vi "Set Password.vi"(8 "error in (no error)":errorcluster, 9 "New password":string, 10 "ProjectItem Refnum":refnum<vi>, 11 "Build in":refnum<class "NI_AB_API_Build.lvclass">) -> (0 "error out":errorcluster, 3 "Build out":refnum<class "NI_AB_API_Build.lvclass">)   [LabVIEW 2020, in "NI_AB_API_Build.lvclass"]
uses:
  <vilib>/AppBuilder/AB_API/Build/NI_AB_API_Build.lvclass
  <vilib>/AppBuilder/AB_API/Build/NI_AB_API_Build.lvclass/NI_AB_API_Build.ctl
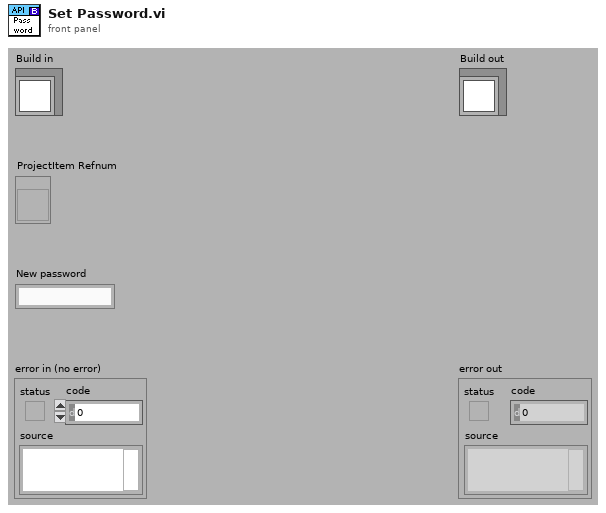
[diagram p1: front panel]
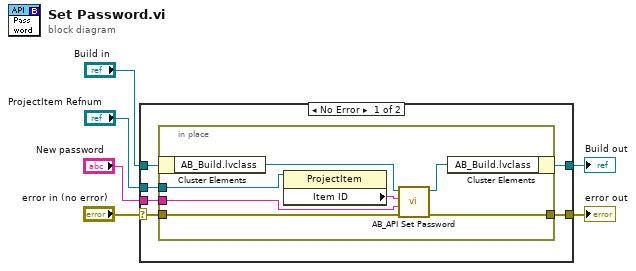
[diagram p0: block diagram]
diagram:
  n1 = case shown="No Error" "error in (no error)" {
    selector: "error in (no error)" -> [w10 w21]
    tunnel: [w11 w21] -> w5
    tunnel: [w7 w20] -> w3
    tunnel: "Build in" -> [w8 w20]
    tunnel: "ProjectItem Refnum" -> [w12 _]
    tunnel: "New password" -> [w9 _]
    frame No Error {
      n2 = in-place {
        in-place-border: w12 -> [w19]
        in-place-border: [w18] -> w11
        in-place-border: w10 -> [w17]
        in-place-border: w9 -> [w16]
        n3 = in-place-cluster #1(w8) -> ("AB_Build.lvclass"=w14:refnum<class "AB_Build.lvclass">)
        n4 = property class="ProjectItem"(reference=w19) -> ("Item ID"=w15:string)  [unwired: 1 in, 2 out]
        n5 = call <vilib>:"AB_API Set Password.vi"("error in (no error)"=w17, "New password"=w16, "source item ID"=w15, "Build in"=w14) -> ("error out"=w18:errorcluster, "Build out"=w13:refnum<class "AB_Build.lvclass">)  [unwired: 6 out]
        n6 = in-place-cluster #1("AB_Build.lvclass"=w13) -> (w7:refnum<class "NI_AB_API_Build.lvclass">)
      }
    }
    frame Error {
    }
  }
  "error out" <- w5
  "Build out" <- w3
